vi "5001.vi"(8 "错误输入（无错误）":errorcluster) -> (0 "error out":errorcluster)   [LabVIEW 2016, in "数据传输系统-05.lvlib"]
uses:
  <vilib>/Utility/config.llb/Read Key (String).vi
  <vilib>/Utility/config.llb/Write Key (String).vi
  <vilib>/Utility/config.llb/NI_LVConfig.lvlib
  <vilib>/ptbypt/NI_PtbyPt.lvlib
panel:
  out "拆分数据":bool
  in  "上传数据类型":string(combo)="在线ADCP分层数据"
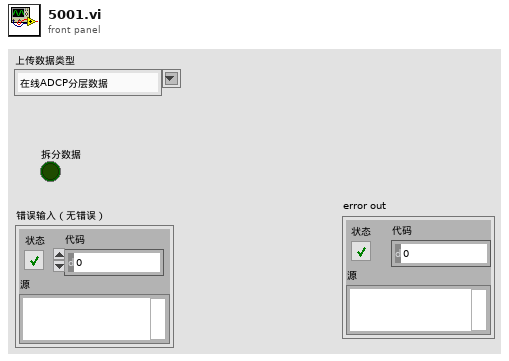
[diagram p1: front panel]
types:
  T1 = cluster{"setini":string, "sysini":string, "hechaini":string, "actualwrite":string, "actualread":string, "datasent":string, "反控命令信息队列":string, "反控与仪器交互":string}
  T2 = typedef "NI_LVConfig.lvlib/Config Data RefNum.ctl" = refnum<k1>
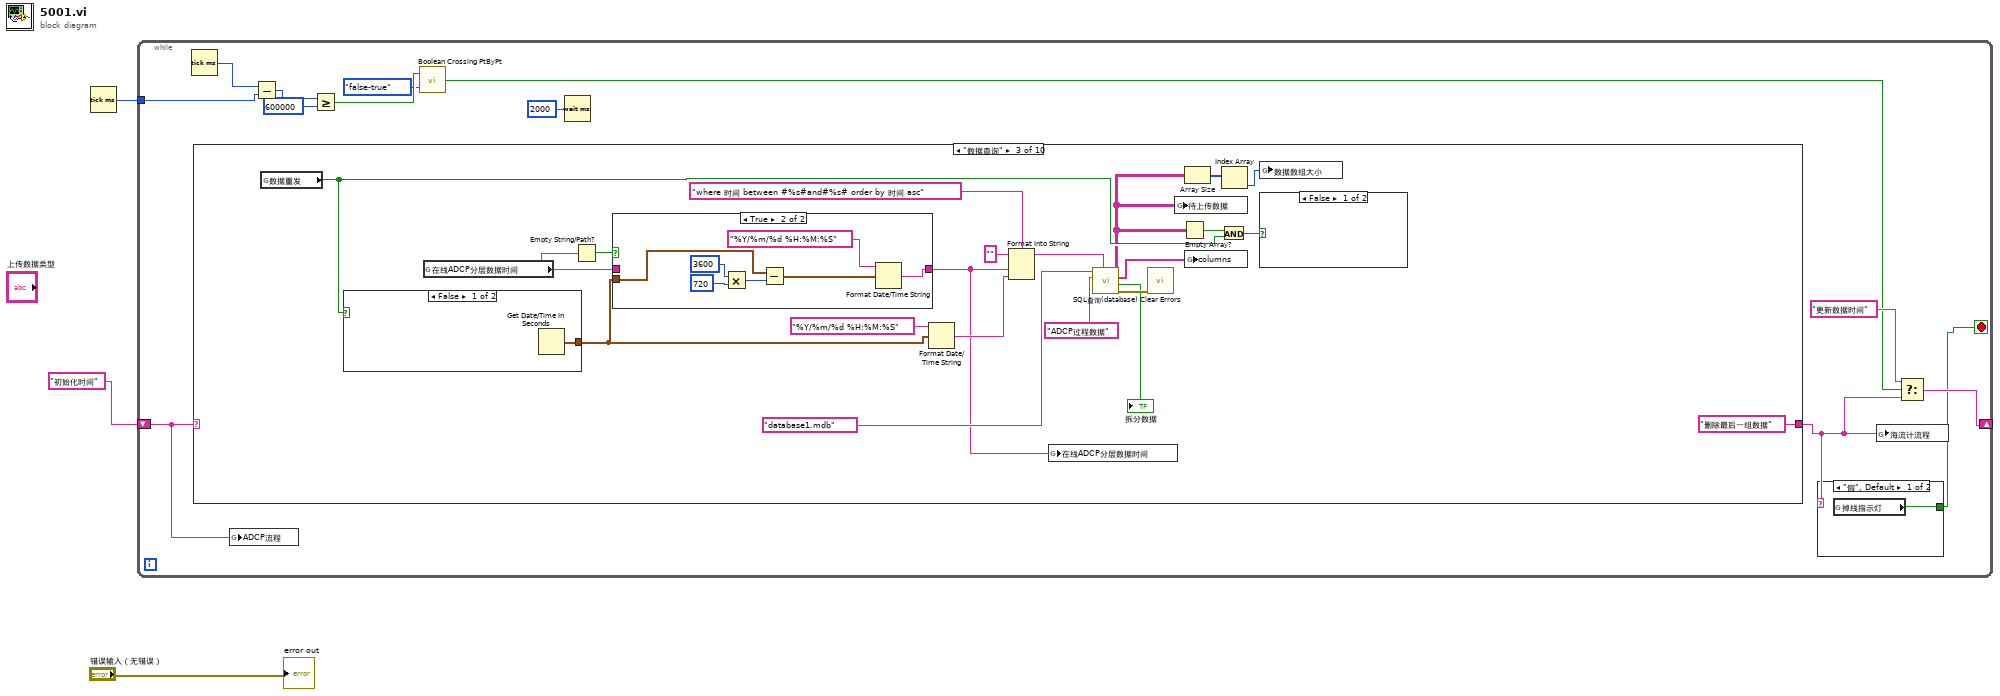
[diagram p0: block diagram]
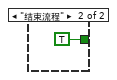
[diagram p2: hidden frame]
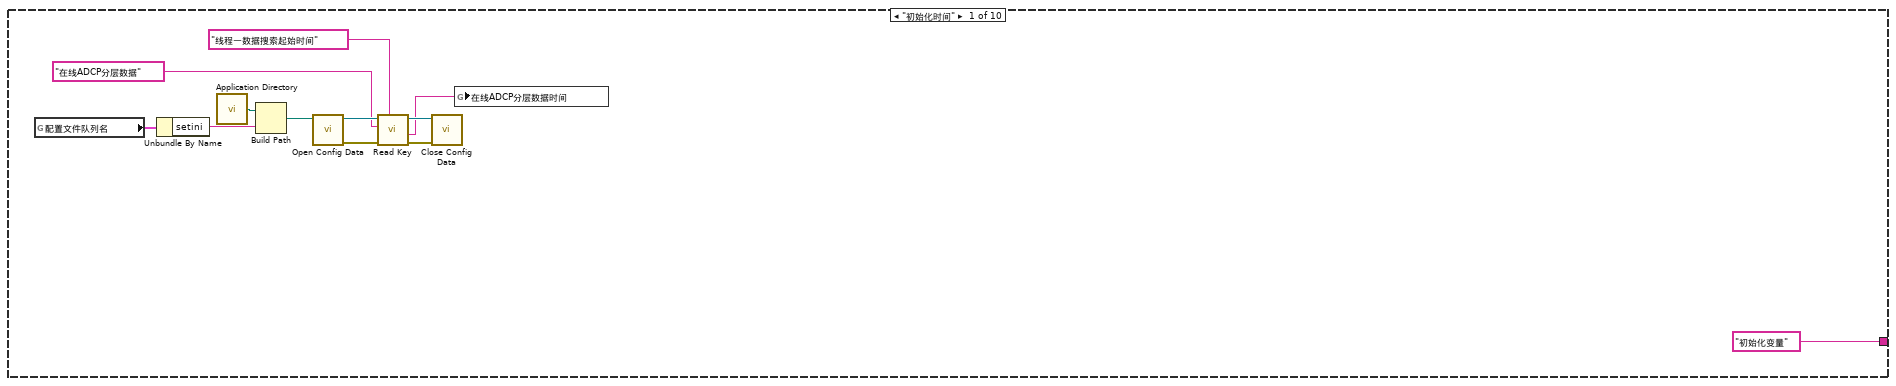
[diagram p3: hidden frame]
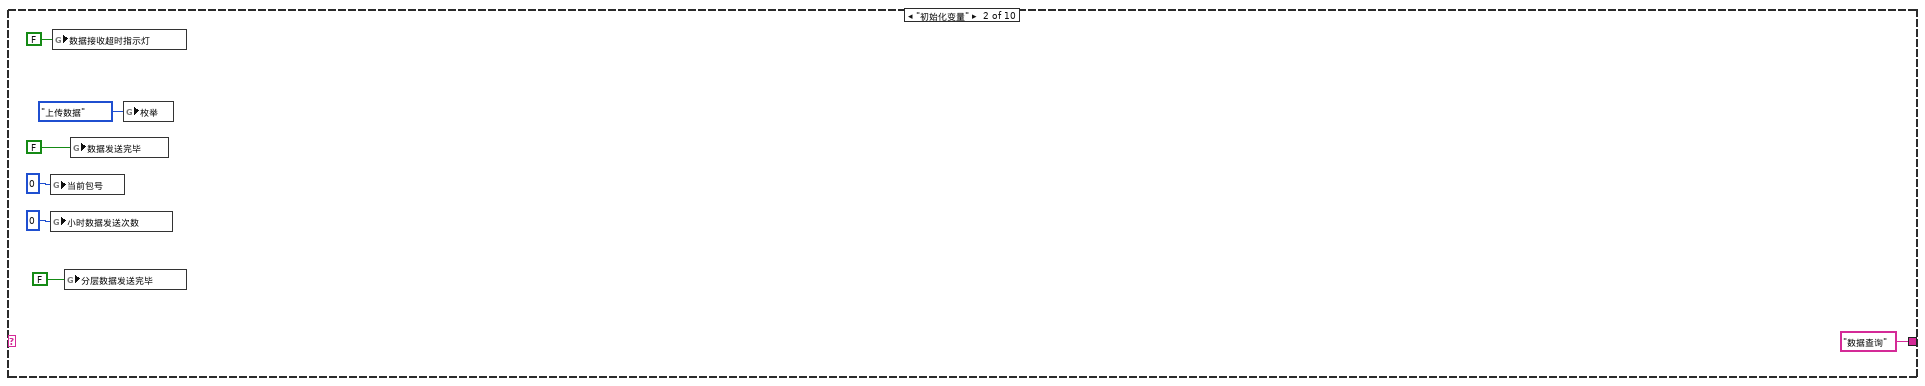
[diagram p4: hidden frame]
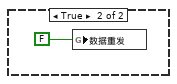
[diagram p5: hidden frame]
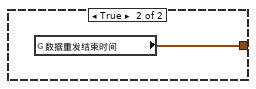
[diagram p7: hidden frame]
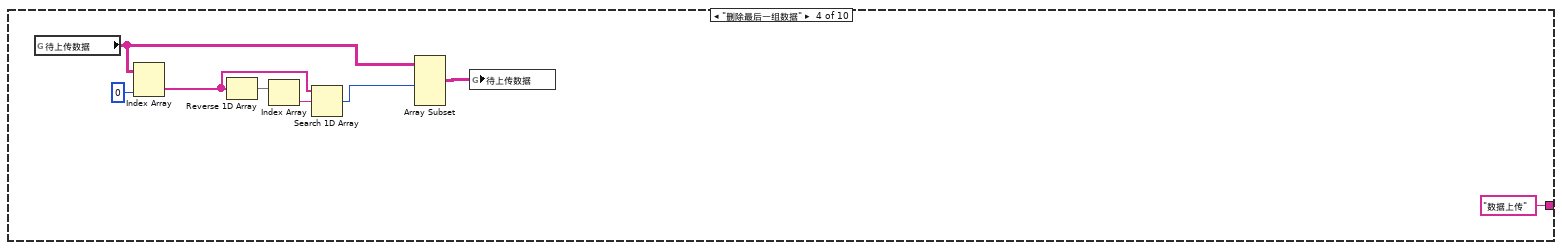
[diagram p8: hidden frame]
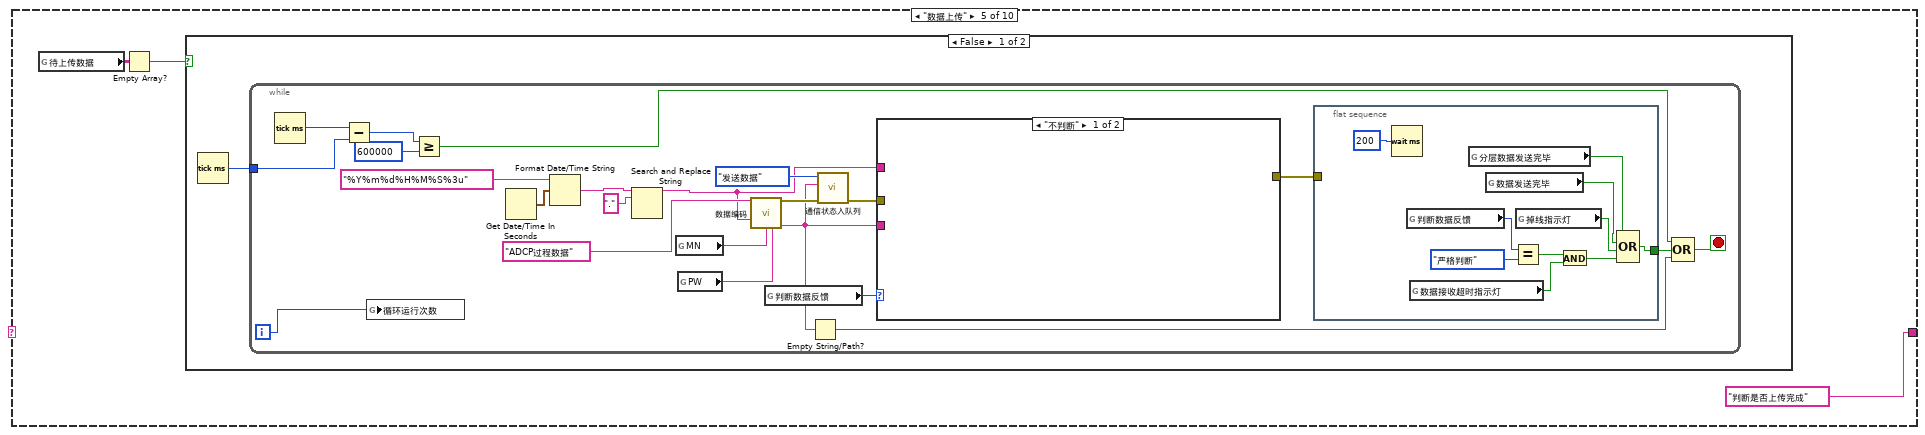
[diagram p9: hidden frame]
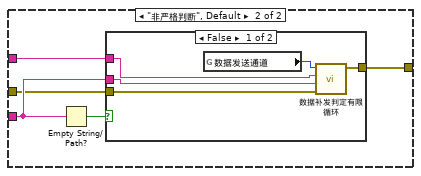
[diagram p10: hidden frame]
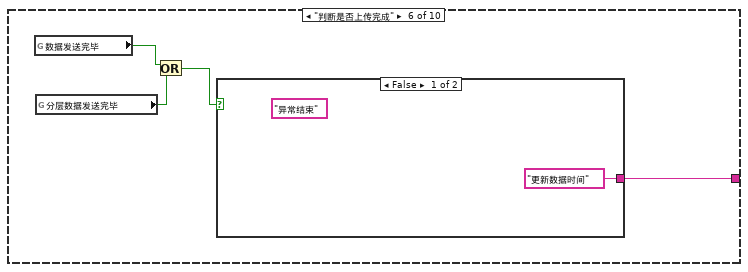
[diagram p13: hidden frame]
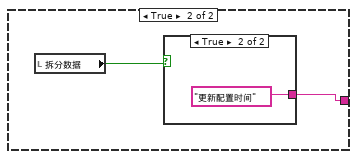
[diagram p14: hidden frame]
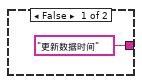
[diagram p15: hidden frame]
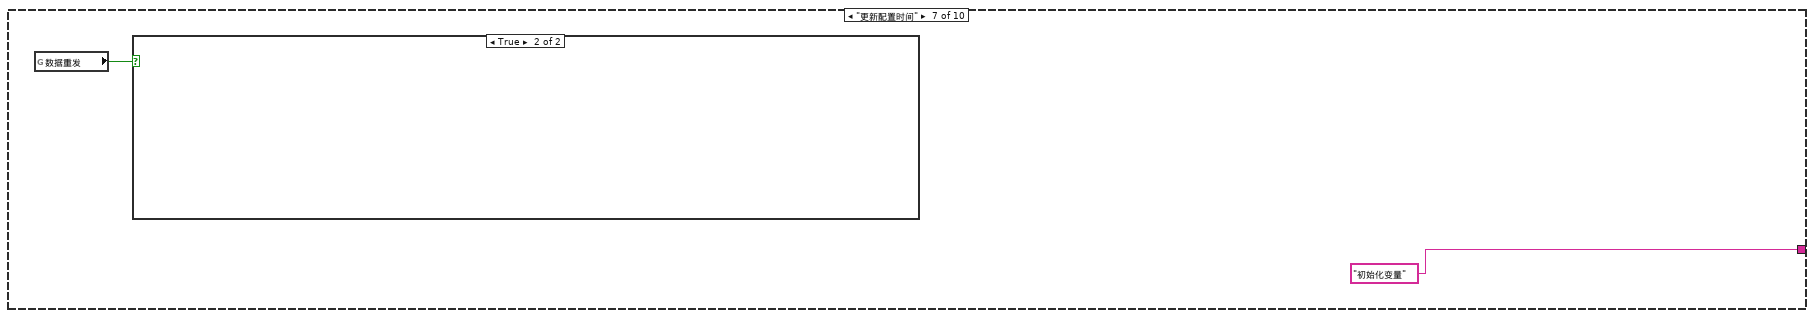
[diagram p16: hidden frame]
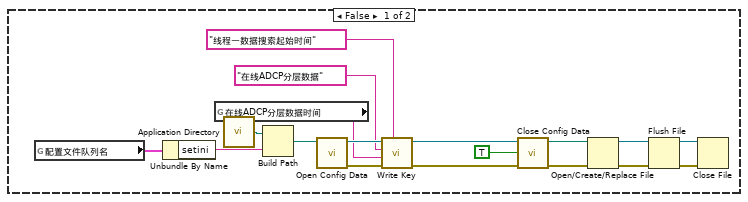
[diagram p17: hidden frame]
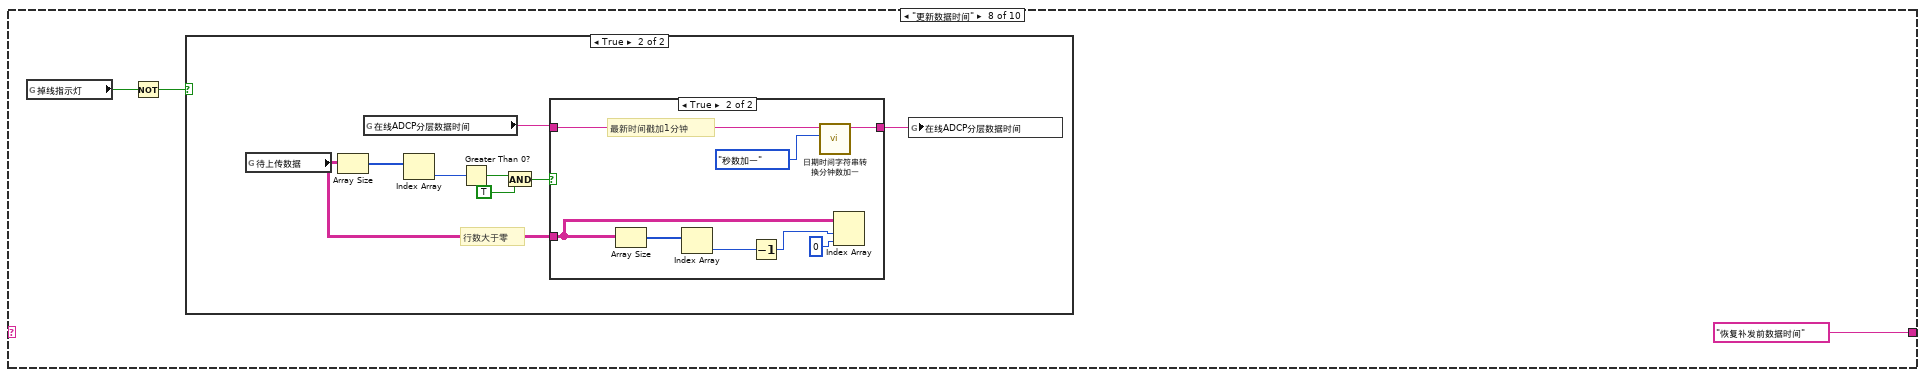
[diagram p18: hidden frame]
diagram:
  n1 = Tick Count (ms)() -> (millisecond timer value=w2:u32)
  n2 = while {
    shift-right: [w11] -> _
    shift-left: "初始化时间" -> [w8]
    tunnel: w2 -> [w15]
    stop <- w10 stop-if-true
    n3 = Tick Count (ms)() -> (millisecond timer value=w16:u32)
    n4 = case shown="\"数据查询\"" w8 {
      tunnel: ["初始化变量" "数据查询" "删除最后一组数据" "数据上传" "判断是否上传完成" w128 "初始化变量" "恢复补发前数据时间" "结束流程" "结束流程"] -> w9
      frame "初始化时间" {
        n5 = global read "全局1.vi" "配置文件队列名"() -> (w30:T1)
        n6 = Unbundle By Name(w30) -> ("setini"=w23:string)
        n7 = call <vilib>:"Application Directory.vi"() -> ("Application Directory"=w24:path)
        n8 = Build Path(base path=w24, name or relative path=w23) -> (appended path=w22:path)
        n9 = call <vilib>:"Open Config Data.vi"("configuration file path"=w22) -> ("error out"=w27:errorcluster, "refnum"=w28:T2)  [unwired: 8 in, 1 out]
        n10 = call-poly <vilib>:"Read Key.vi"("section"="线程一数据搜索起始时间", "error in (no error)"=w27, "key"="在线ADCP分层数据", "refnum"=w28) -> ("error out"=w25:errorcluster, "value"=w21:string, "refnum out"=w26:T2)  [unwired: 4 in, 1 out]
        n11 = call <vilib>:"Close Config Data.vi"("error in (no error)"=w25, "refnum"=w26) -> ()  [unwired: 8 in, 2 out]
        n12 = global write "全局 水样时间.vi" "在线ADCP分层数据时间"(w21) -> ()
      }
      frame "初始化变量" {
        n13 = global write "全局 数据数组大小.vi" "当前包号"(0 ("当前包号")) -> ()
        n14 = global write "全局 小时数据发送次数.vi" "小时数据发送次数"(0 ("小时数据发送次数")) -> ()
        n15 = global write "全局 数据发送重叠.vi" "数据接收超时指示灯"(FALSE ("数据接收超时指示灯")) -> ()
        n16 = global write "全局 数据数组大小.vi" "分层数据发送完毕"(FALSE ("海流计数据发送完毕")) -> ()
        n17 = global write "全局 数据数组大小.vi" "数据发送完毕"(FALSE ("海流计数据发送完毕")) -> ()
        n18 = global write "全局1.vi" "枚举"(enum16{"返回请求应答", "上传数据", "返回执行结果"}."上传数据" ("枚举")) -> ()
      }
      frame "数据查询" {
        n19 = global read "断电保存全局.vi" "数据重发"() -> (w57:bool)
        n20 = case shown="False" w57 {
          tunnel: [w68 w69] -> w52
          frame False {
            n21 = Get Date/Time In Seconds() -> (seconds since 1Jan1904=w68:timestamp)
          }
          frame True {
            n22 = global read "断电保存全局.vi" "数据重发结束时间"() -> (w69:timestamp)
          }
        }
        n23 = global read "全局 水样时间.vi" "在线ADCP分层数据时间"() -> (w53:string)
        n24 = Empty String/Path?(string/path=w53) -> (empty?=w51:bool)
        n25 = case shown="True" w51 {
          tunnel: w52 -> [_ w65]
          tunnel: [w60 w61] -> w38
          tunnel: w53 -> [w60 _]
          frame False {
          }
          frame True {
            n26 = Multiply(x=3600, y=720) -> (x*y=w64:i32)
            n27 = Subtract(x=w65, y=w64) -> (x-y=w62:timestamp)
            n28 = Format Date/Time String(time format string (%c)="%Y/%m/%d %H:%M:%S" ("时间格式字符串(%c)"), seconds (now)=w62) -> (date/time string=w61:string)  [unwired: 1 in]
          }
        }
        n29 = Format Date/Time String(time format string (%c)="%Y/%m/%d %H:%M:%S" ("时间格式字符串(%c)"), seconds (now)=w52) -> (date/time string=w45:string)  [unwired: 1 in]
        n30 = Format Into String(format string="where 时间 between #%s#and#%s# order by 时间 asc" ("condition"), initial string="" ("初始字符串"), w38, w45) -> (resulting string=w46:string)  [unwired: 1 in, 1 out]
        n31 = global write "全局 水样时间.vi" "在线ADCP分层数据时间"(w38) -> ()
        n32 = call "SQL查询(database).vi"("condition"=w46, "table输入"="ADCP过程数据", "database"="database1.mdb") -> ("error out"=w49:errorcluster, "拆分数据"=→"拆分数据":bool, "columns输出"=w54:string[], "data"=w55:string[][])  [unwired: 5 in]
        n33 = call <vilib>:"Clear Errors.vi"("error in (no error)"=w49) -> ()  [unwired: 5 in, 2 out]
        n34 = global write "全局 所有参数.vi" "待上传数据"(w55) -> ()
        n35 = Empty Array?(array=w55) -> (empty?=w56:bool)
        n36 = Array Size(array=w55) -> (size(s)=w47:i32[])
        n37 = global write "全局 所有参数.vi" "columns"(w54) -> ()
        n38 = And(x=w56, y=w57) -> (x .and. y?=w58:bool)
        n39 = Index Array(array=w47) -> (element=w48:i32)  [unwired: 1 in]
        n40 = global write "全局 数据数组大小.vi" "数据数组大小"(w48) -> ()
        n41 = case shown="False" w58 {
          frame False {
          }
          frame True {
            n42 = global write "断电保存全局.vi" "数据重发"(FALSE ("剖面数据重发")) -> ()
          }
        }
      }
      frame "删除最后一组数据" {
        n43 = global read "全局 所有参数.vi" "待上传数据"() -> (w72:string[][])
        n44 = Index Array(array=w72, index (col)=0 ("禁用的索引 (列)")) -> (element=w73:string[])  [unwired: 1 in]
        n45 = Reverse 1D Array(array=w73) -> (reversed array=w75:string[])
        n46 = Index Array(array=w75) -> (element=w74:string)  [unwired: 1 in]
        n47 = Search 1D Array(1D array=w73, element=w74) -> (index of element=w70:i32)  [unwired: 1 in]
        n48 = Array Subset(array=w72, length (row)=w70) -> (w71:string[][])  [unwired: 3 in]
        n49 = global write "全局 所有参数.vi" "待上传数据"(w71) -> ()
      }
      frame "数据上传" {
        n50 = global read "全局 所有参数.vi" "待上传数据"() -> (w79:string[][])
        n51 = Empty Array?(array=w79) -> (empty?=w80:bool)
        n52 = case shown="False" w80 {
          frame False {
            n53 = Tick Count (ms)() -> (millisecond timer value=w81:u32)
            n54 = while {
              tunnel: w81 -> [w88]
              i -> [w82]
              stop <- w86 stop-if-true
              n55 = Tick Count (ms)() -> (millisecond timer value=w89:u32)
              n56 = Subtract(x=w89, y=w88) -> (x-y=w90:u32)
              n57 = global write "全局 水样时间.vi" "循环运行次数"(w82) -> ()
              n58 = Greater Or Equal?(x=w90, y=u32 600000) -> (x >= y?=w85:bool)
              n59 = Get Date/Time In Seconds() -> (seconds since 1Jan1904=w102:timestamp)
              n60 = Format Date/Time String(time format string (%c)="%Y%m%d%H%M%S%3u" ("时间格式字符串(%c)"), seconds (now)=w102) -> (date/time string=w101:string)  [unwired: 1 in]
              n61 = Search and Replace String(input string=w101, search string="." ("搜索字符串")) -> (result string=w94:string)  [unwired: 6 in, 3 out]
              n62 = global read "断电保存全局.vi" "MN"() -> (w96:string)
              n63 = global read "断电保存全局.vi" "PW"() -> (w99:string)
              n64 = call "数据编码.vi"("table输入"="ADCP过程数据" ("新元素/子数组"), "QN"=w94, "MN"=w96, "PW"=w99) -> ("错误常量"=w98:errorcluster, "通讯包字符串"=w84:string)  [unwired: 10 in]
              n65 = global read "断电保存全局.vi" "判断数据反馈"() -> (w93:enum16{"非严格判断", "严格判断", "不判断"})
              n66 = Empty String/Path?(string/path=w84) -> (empty?=w83:bool)
              n67 = call "通信状态入队列.vi"("错误输入（无错误）"=w98, "发送报文"=w84, "枚举"=enum16{"打开连接", "发送数据", "读取数据", "数据处理", "关闭连接"}."发送数据") -> ("错误输出"=w95:errorcluster)  [unwired: 8 in]
              n68 = case shown="\"不判断\"" w93 {
                tunnel: [_ w119] -> w92
                tunnel: w84 -> [_ w118]
                tunnel: w94 -> [_ w117]
                tunnel: w95 -> [_ w115]
                frame "不判断" {
                }
                frame "非严格判断", Default {
                  n69 = Empty String/Path?(string/path=w118) -> (empty?=w116:bool)
                  n70 = case shown="False" w116 {
                    tunnel: [w124 _] -> w119
                    tunnel: w118 -> [w123 _]
                    tunnel: w117 -> [w121 _]
                    tunnel: w115 -> [w120 _]
                    frame False {
                      n71 = global read "断电保存全局.vi" "数据发送通道"() -> (w122:enum16{"TCP", "VISA"})
                      n72 = call "数据补发判定有限循环.vi"("错误输入（无错误）"=w120, "数据输入"=w123, "QN"=w121, "数据发送通道"=w122) -> ("error out"=w124:errorcluster)  [unwired: 7 in]
                    }
                    frame True {
                    }
                  }
                }
              }
              n73 = flat-sequence {
                tunnel: w92 -> [_]
                tunnel: [w109] -> w87
                frame #0 {
                  n74 = Wait (ms)(milliseconds to wait=u32 200 ("等待时间（毫秒）")) -> ()  [unwired: 1 out]
                  n75 = global read "断电保存全局.vi" "判断数据反馈"() -> (w113:enum16{"非严格判断", "严格判断", "不判断"})
                  n76 = global read "全局 数据发送重叠.vi" "数据接收超时指示灯"() -> (w106:bool)
                  n77 = global read "全局 数据数组大小.vi" "分层数据发送完毕"() -> (w105:bool)
                  n78 = global read "全局 数据数组大小.vi" "数据发送完毕"() -> (w108:bool)
                  n79 = Equal?(x=w113, y=enum16{"非严格判断", "严格判断", "不判断"}."严格判断") -> (x = y?=w111:bool)
                  n80 = global read "全局 数据发送重叠.vi" "掉线指示灯"() -> (w107:bool)
                  n81 = And(x=w111, y=w106) -> (x .and. y?=w110:bool)
                  n82 = Compound Arithmetic op=OR ("复合运算")(w105, w108, w107, w110) -> (w109:bool)
                }
              }
              n83 = Compound Arithmetic op=OR ("复合运算")(w85, w87, w83) -> (w86:bool)
            }
          }
          frame True {
          }
        }
      }
      frame "判断是否上传完成" {
        n84 = global read "全局 数据数组大小.vi" "数据发送完毕"() -> (w126:bool)
        n85 = global read "全局 数据数组大小.vi" "分层数据发送完毕"() -> (w127:bool)
        n86 = Or(x=w126, y=w127) -> (x .or. y?=w125:bool)
        n87 = case shown="False" w125 {
          tunnel: ["更新数据时间" w131] -> w128
          frame False {
            (unwired) "异常结束"
          }
          frame True {
            n88 = local read "拆分数据"() -> (w130:bool)
            n89 = case shown="True" w130 {
              tunnel: ["更新数据时间" "更新配置时间"] -> w131
              frame False {
              }
              frame True {
              }
            }
          }
        }
      }
      frame "更新配置时间" {
        n90 = global read "断电保存全局.vi" "数据重发"() -> (w135:bool)
        n91 = case shown="True" w135 {
          frame False {
            n92 = global read "全局1.vi" "配置文件队列名"() -> (w137:T1)
            n93 = Unbundle By Name(w137) -> ("setini"=w138:string)
            n94 = global read "全局 水样时间.vi" "在线ADCP分层数据时间"() -> (w139:string)
            n95 = call <vilib>:"Application Directory.vi"() -> ("Application Directory"=w147:path)
            n96 = Build Path(base path=w147, name or relative path=w138) -> (appended path=w148:path)
            n97 = call <vilib>:"Open Config Data.vi"("configuration file path"=w148) -> ("error out"=w150:errorcluster, "refnum"=w149:T2)  [unwired: 8 in, 1 out]
            n98 = call-poly <vilib>:"Write Key.vi"("section"="线程一数据搜索起始时间", "error in (no error)"=w150, "value"=w139, "key"="在线ADCP分层数据", "refnum"=w149) -> ("error out"=w152:errorcluster, "refnum out"=w151:T2)  [unwired: 4 in, 1 out]
            n99 = call <vilib>:"Close Config Data.vi"("error in (no error)"=w152, "write file if changed (T)"=TRUE, "refnum"=w151) -> ("error out"=w140:errorcluster, "file path"=w141:path)  [unwired: 7 in]
            n100 = Open/Create/Replace File(file path (use dialog)=w141, error in=w140) -> (refnum out=w143:refnum<file>, error out=w142:errorcluster)  [unwired: 4 in, 1 out]
            n101 = Flush File(refnum=w143, error in=w142) -> (refnum out=w144:refnum<file>, error out=w145:errorcluster)
            n102 = Close File(refnum=w144, error in=w145) -> ()  [unwired: 2 out]
          }
          frame True {
          }
        }
      }
      frame "更新数据时间" {
        n103 = global read "全局 数据发送重叠.vi" "掉线指示灯"() -> (w155:bool)
        n104 = Not(x=w155) -> (.not. x?=w156:bool)
        n105 = case shown="True" w156 {
          frame False {
          }
          frame True {
            # "行数大于零"
            n106 = global read "全局 所有参数.vi" "待上传数据"() -> (w163:string[][])
            n107 = Array Size(array=w163) -> (size(s)=w161:i32[])
            n108 = global read "全局 水样时间.vi" "在线ADCP分层数据时间"() -> (w164:string)
            n109 = Index Array(array=w161) -> (element=w162:i32)  [unwired: 1 in]
            n110 = Greater Than 0?(x=w162) -> (x > 0?=w159:bool)
            n111 = And(x=w159, y=TRUE) -> (x .and. y?=w158:bool)
            n112 = case shown="True" w158 {
              tunnel: w163 -> [_ w171]
              tunnel: [w165 w168] -> w160
              tunnel: w164 -> [w165 w167]
              frame False {
              }
              frame True {
                # "最新时间戳加1分钟"
                n113 = Array Size(array=w171) -> (size(s)=w173:i32[])
                n114 = Index Array(array=w173) -> (element=w172:i32)  [unwired: 1 in]
                n115 = Decrement(x=w172) -> (x-1=w170:i32)
                n116 = call "日期时间字符串转换分钟数加一.vi"("枚举"=enum16{"分钟数加一", "秒数加一", "小时数加一"}."秒数加一", "data[0]"=w167) -> ("日期/时间字符串"=w168:string)  [unwired: 9 in]
                n117 = Index Array(array=w171, index (row)=w170, index (col)=0 ("禁用的索引 (列)")) -> ()  [unwired: 1 out]
              }
            }
            n118 = global write "全局 水样时间.vi" "在线ADCP分层数据时间"(w160) -> ()
          }
        }
      }
      frame "恢复补发前数据时间" {
        n119 = global read "断电保存全局.vi" "数据重发"() -> (w175:bool)
        n120 = case shown="False" w175 {
          frame False {
            n121 = global read "全局1.vi" "配置文件队列名"() -> (w177:T1)
            n122 = Unbundle By Name(w177) -> ("setini"=w178:string)
            n123 = global read "全局 水样时间.vi" "在线ADCP分层数据时间"() -> (w179:string)
            n124 = call <vilib>:"Application Directory.vi"() -> ("Application Directory"=w187:path)
            n125 = Build Path(base path=w187, name or relative path=w178) -> (appended path=w188:path)
            n126 = call <vilib>:"Open Config Data.vi"("configuration file path"=w188) -> ("error out"=w190:errorcluster, "refnum"=w189:T2)  [unwired: 8 in, 1 out]
            n127 = call-poly <vilib>:"Write Key.vi"("section"="线程一数据搜索起始时间", "error in (no error)"=w190, "value"=w179, "key"="在线ADCP分层数据", "refnum"=w189) -> ("error out"=w192:errorcluster, "refnum out"=w191:T2)  [unwired: 4 in, 1 out]
            n128 = call <vilib>:"Close Config Data.vi"("error in (no error)"=w192, "write file if changed (T)"=TRUE, "refnum"=w191) -> ("error out"=w180:errorcluster, "file path"=w181:path)  [unwired: 7 in]
            n129 = Open/Create/Replace File(file path (use dialog)=w181, error in=w180) -> (refnum out=w183:refnum<file>, error out=w182:errorcluster)  [unwired: 4 in, 1 out]
            n130 = Flush File(refnum=w183, error in=w182) -> (refnum out=w184:refnum<file>, error out=w185:errorcluster)
            n131 = Close File(refnum=w184, error in=w185) -> ()  [unwired: 2 out]
          }
          frame True {
            n132 = global read "全局1.vi" "配置文件队列名"() -> (w194:T1)
            n133 = global write "断电保存全局.vi" "剖面数据重发"(FALSE ("剖面数据重发")) -> ()
            n134 = Unbundle By Name(w194) -> ("setini"=w202:string)
            n135 = call <vilib>:"Application Directory.vi"() -> ("Application Directory"=w201:path)
            n136 = Build Path(base path=w201, name or relative path=w202) -> (appended path=w203:path)
            n137 = call <vilib>:"Open Config Data.vi"("configuration file path"=w203) -> ("error out"=w198:errorcluster, "refnum"=w197:T2)  [unwired: 8 in, 1 out]
            n138 = call-poly <vilib>:"Read Key.vi"("section"="线程一数据搜索起始时间", "error in (no error)"=w198, "key"="在线ADCP分层数据", "refnum"=w197) -> ("error out"=w200:errorcluster, "value"=w205:string, "refnum out"=w199:T2)  [unwired: 4 in, 1 out]
            n139 = call <vilib>:"Close Config Data.vi"("error in (no error)"=w200, "refnum"=w199) -> ()  [unwired: 8 in, 2 out]
            n140 = global write "全局 水样时间.vi" "在线ADCP分层数据时间"(w205) -> ()
          }
        }
      }
      frame "结束流程", Default {
      }
    }
    n141 = global write "全局 水样时间.vi" "ADCP流程"(w8) -> ()
    n142 = Subtract(x=w16, y=w15) -> (x-y=w14:u32)
    n143 = Greater Or Equal?(x=w14, y=u32 600000) -> (x >= y?=w7:bool)
    n144 = call <vilib>:"Boolean Crossing PtByPt.vi"("direction"=enum16{"either", "false-true", "true-false"}."false-true", "input"=w7) -> ("crossing"=w5:bool)  [unwired: 1 in]
    n145 = Wait (ms)(milliseconds to wait=u32 2000 ("等待时间（毫秒）")) -> ()  [unwired: 1 out]
    n146 = case shown="\"假\", Default" w9 {
      tunnel: [w17 TRUE] -> w10
      frame "假", Default {
        n147 = global read "全局 数据发送重叠.vi" "掉线指示灯"() -> (w17:bool)
      }
      frame "结束流程" {
      }
    }
    n148 = global write "全局 水样时间.vi" "海流计流程"(w9) -> ()
    n149 = Select(t="更新数据时间", s=w5, f=w9) -> (s? t:f=w11:string)
  }
  "error out" <- "错误输入（无错误）"
